vi "Weather Parse Test.vi"() -> ()   [LabVIEW 2020, in "CDM-Config.lvlib"] (continued)
    \"onset\": \"2025-12-03T00:00:00-08:00\",\n                \"expires\": \"2025-12-03T09:00:00-08:00\",\n                \"ends\": \"2025-12-03T09:00:00-08:00\",\n                \"status\": \"Actual\",\n                \"messageType\": \"Update\",\n                \"category\": \"Met\",\n                \"severity\": \"Minor\",\n                \"certainty\": \"Likely\",\n                \"urgency\": \"Expected\",\n                \"event\": \"Frost Advisory\",\n                \"sender\": \"w-nws.webmaster@noaa.gov\",\n                \"senderName\": \"NWS Eureka CA\",\n                \"headline\": \"Frost Advisory issued December 2 at 6:17PM PST until December 3 at 9:00AM PST by NWS Eureka CA\",\n                \"description\": \"* WHAT...Temperatures as low as 33 will result in frost formation.\\n\\n* WHERE...Humboldt Interior.\\n\\n* WHEN...From midnight tonight to 9 AM PST Wednesday.\\n\\n* IMPACTS...Frost could harm sensitive outdoor vegetation. Sensitive\\noutdoor plants may be killed if left uncovered.\\n\\n* ADDITIONAL DETAILS...Fog or low clouds may develop in some valleys\\nkeeping temperatures in the upper 30s.\",\n                \"instruction\": \"Take steps now to protect tender plants from the cold.\",\n                \"response\": \"Prepare\",\n                \"parameters\": {\n                    \"AWIPSidentifier\": [\n                        \"NPWEKA\"\n                    ],\n                    \"WMOidentifier\": [\n                        \"WWUS76 KEKA 030217\"\n                    ],\n                    \"NWSheadline\": [\n                        \"FROST ADVISORY REMAINS IN EFFECT FROM MIDNIGHT TONIGHT TO 9 AM PST WEDNESDAY\"\n                    ],\n                    \"BLOCKCHANNEL\": [\n                        \"EAS\",\n                        \"NWEM\",\n                        \"CMAS\"\n                    ],\n                    \"VTEC\": [\n                        \"/O.CON.KEKA.FR.Y.0037.251203T0800Z-251203T1700Z/\"\n                    ],\n                    \"eventEndingTime\": [\n                        \"2025-12-03T09:00:00-08:00\"\n                    ]\n                },\n                \"scope\": \"Public\",\n                \"code\": \"IPAWSv1.0\",\n                \"language\": \"en-US\",\n                \"web\": \"http://www.weather.gov\",\n                \"eventCode\": {\n                    \"SAME\": [\n                        \"NWS\"\n                    ],\n                    \"NationalWeatherService\": [\n                        \"FRY\"\n                    ]\n                }\n            }\n        },\n        {\n            \"id\": \"https://api.weather.gov/alerts/urn:oid:2.49.0.1.840.0.9a5af99817b4d9edcfcd61f0327d754f8de44e19.004.1\",\n            \"type\": \"Feature\",\n            \"geometry\": null,\n            \"properties\": {\n                \"@id\": \"https://api.weather.gov/alerts/urn:oid:2.49.0.1.840.0.9a5af99817b4d9edcfcd61f0327d754f8de44e19.004.1\",\n                \"@type\": \"wx:Alert\",\n                \"id\": \"urn:oid:2.49.0.1.840.0.9a5af99817b4d9edcfcd61f0327d754f8de44e19.004.1\",\n                \"areaDesc\": \"Southwestern Mendocino Interior; Southeastern Mendocino Interior\",\n                \"geocode\": {\n                    \"SAME\": [\n                        \"006045\"\n                    ],\n                    \"UGC\": [\n                        \"CAZ112\",\n                        \"CAZ113\"\n                    ]\n                },\n                \"affectedZones\": [\n                    \"https://api.weather.gov/zones/forecast/CAZ112\",\n                    \"https://api.weather.gov/zones/forecast/CAZ113\"\n                ],\n                \"references\": [\n                    {\n                        \"@id\": \"https://api.weather.gov/alerts/urn:oid:2.49.0.1.840.0.95406e8f32c287b077c961d659d14abba87dc6d0.003.1\",\n                        \"identifier\": \"urn:oid:2.49.0.1.840.0.95406e8f32c287b077c961d659d14abba87dc6d0.003.1\",\n                        \"sender\": \"w-nws.webmaster@noaa.gov\",\n                        \"sent\": \"2025-12-02T10:21:00-08:00\"\n                    },\n                    {\n                        \"@id\": \"https://api.weather.gov/alerts/urn:oid:2.49.0.1.840.0.572af28717b4d18ac951aaf092ab1eb478907437.004.1\",\n                        \"identifier\": \"urn:oid:2.49.0.1.840.0.572af28717b4d18ac951aaf092ab1eb478907437.004.1\",\n                        \"sender\": \"w-nws.webmaster@noaa.gov\",\n                        \"sent\": \"2025-12-02T10:26:00-08:00\"\n                    }\n                ],\n                \"sent\": \"2025-12-02T18:17:00-08:00\",\n                \"effective\": \"2025-12-02T18:17:00-08:00\",\n                \"onset\": \"2025-12-03T00:00:00-08:00\",\n                \"expires\": \"2025-12-03T09:00:00-08:00\",\n                \"ends\": \"2025-12-03T09:00:00-08:00\",\n                \"status\": \"Actual\",\n                \"messageType\": \"Update\",\n                \"category\": \"Met\",\n                \"severity\": \"Minor\",\n                \"certainty\": \"Likely\",\n                \"urgency\": \"Expected\",\n                \"event\": \"Frost Advisory\",\n                \"sender\": \"w-nws.webmaster@noaa.gov\",\n                \"senderName\": \"NWS Eureka CA\",\n                \"headline\": \"Frost Advisory issued December 2 at 6:17PM PST until December 3 at 9:00AM PST by NWS Eureka CA\",\n                \"description\": \"* WHAT...Temperatures as low as 34 will result in frost formation.\\n\\n* WHERE...Southern Mendocino Interior valleys.\\n\\n* WHEN...From midnight tonight to 9 AM PST Wednesday.\\n\\n* IMPACTS...Frost could harm sensitive outdoor vegetation. Sensitive\\noutdoor plants may be killed if left uncovered.\\n\\n* ADDITIONAL DETAILS...Fog or low clouds may develop in some valleys\\nkeeping temperatures in the upper 30s.\",\n                \"instruction\": \"Take steps now to protect tender plants from the cold.\",\n                \"response\": \"Prepare\",\n                \"parameters\": {\n                    \"AWIPSidentifier\": [\n                        \"NPWEKA\"\n                    ],\n                    \"WMOidentifier\": [\n                        \"WWUS76 KEKA 030217\"\n                    ],\n                    \"NWSheadline\": [\n                        \"FROST ADVISORY REMAINS IN EFFECT FROM MIDNIGHT TONIGHT TO 9 AM PST WEDNESDAY\"\n                    ],\n                    \"BLOCKCHANNEL\": [\n                        \"EAS\",\n                        \"NWEM\",\n                        \"CMAS\"\n                    ],\n                    \"VTEC\": [\n                        \"/O.CON.KEKA.FR.Y.0037.251203T0800Z-251203T1700Z/\"\n                    ],\n                    \"eventEndingTime\": [\n                        \"2025-12-03T09:00:00-08:00\"\n                    ]\n                },\n                \"scope\": \"Public\",\n                \"code\": \"IPAWSv1.0\",\n                \"language\": \"en-US\",\n                \"web\": \"http://www.weather.gov\",\n                \"eventCode\": {\n                    \"SAME\": [\n                        \"NWS\"\n                    ],\n                    \"NationalWeatherService\": [\n                        \"FRY\"\n                    ]\n                }\n            }\n        },\n        {\n            \"id\": \"https://api.weather.gov/alerts/urn:oid:2.49.0.1.840.0.9a5af99817b4d9edcfcd61f0327d754f8de44e19.001.1\",\n            \"type\": \"Feature\",\n            \"geometry\": null,\n            \"properties\": {\n                \"@id\": \"https://api.weather.gov/alerts/urn:oid:2.49.0.1.840.0.9a5af99817b4d9edcfcd61f0327d754f8de44e19.001.1\",\n                \"@type\": \"wx:Alert\",\n                \"id\": \"urn:oid:2.49.0.1.840.0.9a5af99817b4d9edcfcd61f0327d754f8de44e19.001.1\",\n                \"areaDesc\": \"Northern Humboldt Coast; Southwestern Humboldt\",\n                \"geocode\": {\n                    \"SAME\": [\n                        \"006023\"\n                    ],\n                    \"UGC\": [\n                        \"CAZ103\",\n                        \"CAZ104\"\n                    ]\n                },\n                \"affectedZones\": [\n                    \"https://api.weather.gov/zones/forecast/CAZ103\",\n                    \"https://api.weather.gov/zones/forecast/CAZ104\"\n                ],\n                \"references\": [\n                    {\n                        \"@id\": \"https://api.weather.gov/alerts/urn:oid:2.49.0.1.840.0.95406e8f32c287b077c961d659d14abba87dc6d0.001.1\",\n                        \"identifier\": \"urn:oid:2.49.0.1.840.0.95406e8f32c287b077c961d659d14abba87dc6d0.001.1\",\n                        \"sender\": \"w-nws.webmaster@noaa.gov\",\n                        \"sent\": \"2025-12-02T10:21:00-08:00\"\n                    },\n                    {\n                        \"@id\": \"https://api.weather.gov/alerts/urn:oid:2.49.0.1.840.0.572af28717b4d18ac951aaf092ab1eb478907437.002.1\",\n                        \"identifier\": \"urn:oid:2.49.0.1.840.0.572af28717b4d18ac951aaf092ab1eb478907437.002.1\",\n                        \"sender\": \"w-nws.webmaster@noaa.gov\",\n                        \"sent\": \"2025-12-02T10:26:00-08:00\"\n                    }\n                ],\n                \"sent\": \"2025-12-02T18:17:00-08:00\",\n                \"effective\": \"2025-12-02T18:17:00-08:00\",\n                \"onset\": \"2025-12-03T00:00:00-08:00\",\n                \"expires\": \"2025-12-03T09:00:00-08:00\",\n                \"ends\": \"2025-12-03T09:00:00-08:00\",\n                \"status\": \"Actual\",\n                \"messageType\": \"Update\",\n                \"category\": \"Met\",\n                \"severity\": \"Minor\",\n                \"certainty\": \"Likely\",\n                \"urgency\": \"Expected\",\n                \"event\": \"Frost Advisory\",\n                \"sender\": \"w-nws.webmaster@noaa.gov\",\n                \"senderName\": \"NWS Eureka CA\",\n                \"headline\": \"Frost Advisory issued December 2 at 6:17PM PST until December 3 at 9:00AM PST by NWS Eureka CA\",\n                \"description\": \"* WHAT...Temperatures as low as 34 will result in frost formation.\\n\\n* WHERE...Humboldt Coast.\\n\\n* WHEN...From midnight tonight to 9 AM PST Wednesday.\\n\\n* IMPACTS...Frost could harm sensitive outdoor vegetation. Sensitive\\noutdoor plants may be killed if left uncovered.\\n\\n* ADDITIONAL DETAILS...Coldest areas will be valleys that remain\\nclear and are away from the coast.\",\n                \"instruction\": \"Take steps now to protect tender plants from the cold.\",\n                \"response\": \"Prepare\",\n                \"parameters\": {\n                    \"AWIPSidentifier\": [\n                        \"NPWEKA\"\n                    ],\n                    \"WMOidentifier\": [\n                        \"WWUS76 KEKA 030217\"\n                    ],\n                    \"NWSheadline\": [\n                        \"FROST ADVISORY REMAINS IN EFFECT FROM MIDNIGHT TONIGHT TO 9 AM PST WEDNESDAY\"\n                    ],\n                    \"BLOCKCHANNEL\": [\n                        \"EAS\",\n                        \"NWEM\",\n                        \"CMAS\"\n                    ],\n                    \"VTEC\": [\n                        \"/O.CON.KEKA.FR.Y.0037.251203T0800Z-251203T1700Z/\"\n                    ],\n                    \"eventEndingTime\": [\n                        \"2025-12-03T09:00:00-08:00\"\n                    ]\n                },\n                \"scope\": \"Public\",\n                \"code\": \"IPAWSv1.0\",\n                \"language\": \"en-US\",\n                \"web\": \"http://www.weather.gov\",\n                \"eventCode\": {\n                    \"SAME\": [\n                        \"NWS\"\n                    ],\n                    \"NationalWeatherService\": [\n                        \"FRY\"\n                    ]\n                }\n            }\n        },\n        {\n            \"id\": \"https://api.weather.gov/alerts/urn:oid:2.49.0.1.840.0.9a5af99817b4d9edcfcd61f0327d754f8de44e19.003.1\",\n            \"type\": \"Feature\",\n            \"geometry\": null,\n            \"properties\": {\n                \"@id\": \"https://api.weather.gov/alerts/urn:oid:2.49.0.1.840.0.9a5af99817b4d9edcfcd61f0327d754f8de44e19.003.1\",\n                \"@type\": \"wx:Alert\",\n                \"id\": \"urn:oid:2.49.0.1.840.0.9a5af99817b4d9edcfcd61f0327d754f8de44e19.003.1\",\n                \"areaDesc\": \"Mendocino Coast\",\n                \"geocode\": {\n                    \"SAME\": [\n                        \"006045\"\n                    ],\n                    \"UGC\": [\n                        \"CAZ109\"\n                    ]\n                },\n                \"affectedZones\": [\n                    \"https://api.weather.gov/zones/forecast/CAZ109\"\n                ],\n                \"references\": [\n                    {\n                        \"@id\": \"https://api.weather.gov/alerts/urn:oid:2.49.0.1.840.0.95406e8f32c287b077c961d659d14abba87dc6d0.002.1\",\n                        \"identifier\": \"urn:oid:2.49.0.1.840.0.95406e8f32c287b077c961d659d14abba87dc6d0.002.1\",\n                        \"sender\": \"w-nws.webmaster@noaa.gov\",\n                        \"sent\": \"2025-12-02T10:21:00-08:00\"\n                    },\n                    {\n                        \"@id\": \"https://api.weather.gov/alerts/urn:oid:2.49.0.1.840.0.572af28717b4d18ac951aaf092ab1eb478907437.003.1\",\n                        \"identifier\": \"urn:oid:2.49.0.1.840.0.572af28717b4d18ac951aaf092ab1eb478907437.003.1\",\n                        \"sender\": \"w-nws.webmaster@noaa.gov\",\n                        \"sent\": \"2025-12-02T10:26:00-08:00\"\n                    }\n                ],\n                \"sent\": \"2025-12-02T18:17:00-08:00\",\n                \"effective\": \"2025-12-02T18:17:00-08:00\",\n                \"onset\": \"2025-12-03T00:00:00-08:00\",\n                \"expires\": \"2025-12-03T09:00:00-08:00\",\n                \"ends\": \"2025-12-03T09:00:00-08:00\",\n                \"status\": \"Actual\",\n                \"messageType\": \"Update\",\n                \"category\": \"Met\",\n                \"severity\": \"Minor\",\n                \"certainty\": \"Likely\",\n                \"urgency\": \"Expected\",\n                \"event\": \"Frost Advisory\",\n                \"sender\": \"w-nws.webmaster@noaa.gov\",\n                \"senderName\": \"NWS Eureka CA\",\n                \"headline\": \"Frost Advisory issued December 2 at 6:17PM PST until December 3 at 9:00AM PST by NWS Eureka CA\",\n                \"description\": \"* WHAT...Temperatures as low as 34 will result in frost formation.\\n\\n* WHERE...Mendocino Coast. The coldest areas will be just inland from\\nthe coast.\\n\\n* WHEN...From midnight tonight to 9 AM PST Wednesday.\\n\\n* IMPACTS...Frost could harm sensitive outdoor vegetation. Sensitive\\noutdoor plants may be killed if left uncovered.\",\n                \"instruction\": \"Take steps now to protect tender plants from the cold.\",\n                \"response\": \"Prepare\",\n                \"parameters\": {\n                    \"AWIPSidentifier\": [\n                        \"NPWEKA\"\n                    ],\n                    \"WMOidentifier\": [\n                        \"WWUS76 KEKA 030217\"\n                    ],\n                    \"NWSheadline\": [\n                        \"FROST ADVISORY REMAINS IN EFFECT FROM MIDNIGHT TONIGHT TO 9 AM PST WEDNESDAY\"\n                    ],\n                    \"BLOCKCHANNEL\": [\n                        \"EAS\",\n                        \"NWEM\",\n                        \"CMAS\"\n                    ],\n                    \"VTEC\": [\n                        \"/O.CON.KEKA.FR.Y.0037.251203T0800Z-251203T1700Z/\"\n                    ],\n                    \"eventEndingTime\": [\n                        \"2025-12-03T09:00:00-08:00\"\n                    ]\n                },\n                \"scope\": \"Public\",\n                \"code\": \"IPAWSv1.0\",\n                \"language\": \"en-US\",\n                \"web\": \"http://www.weather.gov\",\n                \"eventCode\": {\n                    \"SAME\": [\n                        \"NWS\"\n                    ],\n                    \"NationalWeatherService\": [\n                        \"FRY\"\n                    ]\n                }\n            }\n        },\n        {\n            \"id\": \"https://api.weather.gov/alerts/urn:oid:2.49.0.1.840.0.90d765b84bbb08e28d74a226f4e1f9e6e65de885.006.1\",\n            \"type\": \"Feature\",\n            \"geometry\": null,\n            \"properties\": {\n                \"@id\": \"https://api.weather.gov/alerts/urn:oid:2.49.0.1.840.0.90d765b84bbb08e28d74a226f4e1f9e6e65de885.006.1\",\n                \"@type\": \"wx:Alert\",\n                \"id\": \"urn:oid:2.49.0.1.840.0.90d765b84bbb08e28d74a226f4e1f9e6e65de885.006.1\",\n                \"areaDesc\": \"Cape Tolstoi to Cape Sarichef out to 15 NM\",\n                \"geocode\": {\n                    \"SAME\": [\n                        \"058754\"\n                    ],\n                    \"UGC\": [\n                        \"PKZ754\"\n                    ]\n                },\n                \"affectedZones\": [\n                    \"https://api.weather.gov/zones/forecast/PKZ754\"\n                ],\n                \"references\": [],\n                \"sent\": \"2025-12-02T16:08:00-09:00\",\n                \"effective\": \"2025-12-02T16:08:00-09:00\",\n                \"onset\": \"2025-12-03T05:00:00-09:00\",\n                \"expires\": \"2025-12-03T05:15:00-09:00\",\n                \"ends\": \"2025-12-04T05:00:00-09:00\",\n                \"status\": \"Actual\",\n                \"messageType\": \"Alert\",\n                \"category\": \"Met\",\n                \"severity\": \"Minor\",\n                \"certainty\": \"Likely\",\n                \"urgency\": \"Expected\",\n                \"event\": \"Small Craft Advisory\",\n                \"sender\": \"w-nws.webmaster@noaa.gov\",\n                \"senderName\": \"NWS Anchorage AK\",\n                \"headline\": \"Small Craft Advisory issued December 2 at 4:08PM AKST until December 4 at 5:00AM AKST by NWS Anchorage AK\",\n                \"description\": \"Coastal Waters Forecast for Southwest Alaska+Bristol Bay+The\\nAlaska Peninsula Waters and the Aleutian Islands up to 100 nm out.\\n\\nWind forecasts reflect the predominant speed and direction\\nexpected. Sea forecasts represent an average of the highest\\none-third of the combined wind wave and swell height.\\n\\n.TONIGHT...SE wind 30 kt. Seas 18 ft. Rain.\\n.WED...SE wind 25 kt. Seas 13 ft. Rain.\\n.WED NIGHT...SE wind 15 kt. Seas 11 ft. Rain.\\n.THU AND THU NIGHT...NE wind 15 kt. Seas 7 ft.\\n.FRI...N wind 25 kt. Seas 5 ft.\\n.SAT...NW wind 35 kt. Seas 6 ft.\\n.SUN...N wind 25 kt. Seas 5 ft.\",\n                \"instruction\": null,\n                \"response\": \"Avoid\",\n                \"parameters\": {\n                    \"AWIPSidentifier\": [\n                        \"CWFALU\"\n                    ],\n                    \"WMOidentifier\": [\n                        \"FZAK52 PAFC 030108\"\n                    ],\n                    \"NWSheadline\": [\n                        \"SMALL CRAFT ADVISORY THROUGH WEDNESDAY NIGHT\"\n                    ],\n                    \"BLOCKCHANNEL\": [\n                        \"EAS\",\n                        \"NWEM\",\n                        \"CMAS\"\n                    ],\n                    \"VTEC\": [\n                        \"/O.NEW.PAFC.SC.Y.9898.251203T1400Z-251204T1400Z/\"\n                    ],\n                    \"eventEndingTime\": [\n                        \"2025-12-04T05:00:00-09:00\"\n                    ]\n                },\n                \"scope\": \"Public\",\n                \"code\": \"IPAWSv1.0\",\n                \"language\": \"en-US\",\n                \"web\": \"http://www.weather.gov\",\n                \"eventCode\": {\n                    \"SAME\": [\n                        \"NWS\"\n                    ],\n                    \"NationalWeatherService\": [\n                        \"SCY\"\n                    ]\n                }\n            }\n        },\n        {\n            \"id\": \"https://api.weather.gov/alerts/urn:oid:2.49.0.1.840.0.90d765b84bbb08e28d74a226f4e1f9e6e65de885.003.1\",\n            \"type\": \"Feature\",\n            \"geometry\": null,\n            \"properties\": {\n                \"@id\": \"https://api.weather.gov/alerts/urn:oid:2.49.0.1.840.0.90d765b84bbb08e28d74a226f4e1f9e6e65de885.003.1\",\n                \"@type\": \"wx:Alert\",\n                \"id\": \"urn:oid:2.49.0.1.840.0.90d765b84bbb08e28d74a226f4e1f9e6e65de885.003.1\",\n                \"areaDesc\": \"Sitkinak to Castle Cape from 15 to 100 NM\",\n                \"geocode\": {\n                    \"SAME\": [\n                        \"058751\"\n                    ],\n                    \"UGC\": [\n                        \"PKZ751\"\n                    ]\n                },\n                \"affectedZones\": [\n                    \"https://api.weather.gov/zones/forecast/PKZ751\"\n                ],\n                \"references\": [],\n                \"sent\": \"2025-12-02T16:08:00-09:00\",\n                \"effective\": \"2025-12-02T16:08:00-09:00\",\n                \"onset\": \"2025-12-03T05:00:00-09:00\",\n                \"expires\": \"2025-12-03T05:15:00-09:00\",\n                \"ends\": \"2025-12-04T05:00:00-09:00\",\n                \"status\": \"Actual\",\n                \"messageType\": \"Alert\",\n                \"category\": \"Met\",\n                \"severity\": \"Minor\",\n                \"certainty\": \"Likely\",\n                \"urgency\": \"Expected\",\n                \"event\": \"Small Craft Advisory\",\n                \"sender\": \"w-nws.webmaster@noaa.gov\",\n                \"senderName\": \"NWS Anchorage AK\",\n                \"headline\": \"Small Craft Advisory issued December 2 at 4:08PM AKST until December 4 at 5:00AM AKST by NWS Anchorage AK\",\n                \"description\": \"Coastal Waters Forecast for Southwest Alaska+Bristol Bay+The\\nAlaska Peninsula Waters and the Aleutian Islands up to 100 nm out.\\n\\nWind forecasts reflect the predominant speed and direction\\nexpected. Sea forecasts represent an average of the highest\\none-third of the combined wind wave and swell height.\\n\\n.TONIGHT...SE wind 25 kt. Seas 17 ft.\\n.WED...S wind 20 kt. Seas 14 ft.\\n.WED NIGHT...S wind 20 kt. Seas 14 ft.\\n.THU...E wind 20 kt. Seas 12 ft.\\n.THU NIGHT...E wind 30 kt. Seas 10 ft.\\n.FRI THROUGH SAT...NW wind 35 kt. Seas 10 ft.\\n.SUN...N wind 25 kt. Seas 9 ft.\",\n                \"instruction\": null,\n                \"response\": \"Avoid\",\n                \"parameters\": {\n                    \"AWIPSidentifier\": [\n                        \"CWFALU\"\n                    ],\n                    \"WMOidentifier\": [\n                        \"FZAK52 PAFC 030108\"\n                    ],\n                    \"NWSheadline\": [\n                        \"SMALL CRAFT ADVISORY THROUGH WEDNESDAY NIGHT\"\n                    ],\n                    \"BLOCKCHANNEL\": [\n                        \"EAS\",\n                        \"NWEM\",\n                        \"CMAS\"\n                    ],\n                    \"VTEC\": [\n                        \"/O.NEW.PAFC.SC.Y.9895.251203T1400Z-251204T1400Z/\"\n                    ],\n                    \"eventEndingTime\": [\n                        \"2025-12-04T05:00:00-09:00\"\n                    ]\n                },\n                \"scope\": \"Public\",\n                \"code\": \"IPAWSv1.0\",\n                \"language\": \"en-US\",\n                \"web\": \"http://www.weather.gov\",\n                \"eventCode\": {\n                    \"SAME\": [\n                        \"NWS\"\n                    ],\n                    \"NationalWeatherService\": [\n                        \"SCY\"\n                    ]\n                }\n            }\n        },\n        {\n            \"id\": \"https://api.weather.gov/alerts/urn:oid:2.49.0.1.840.0.90d765b84bbb08e28d74a226f4e1f9e6e65de885.007.1\",\n            \"type\": \"Feature\",\n            \"geometry\": null,\n            \"properties\": {\n                \"@id\": \"https://api.weather.gov/alerts/urn:oid:2.49.0.1.840.0.90d765b84bbb08e28d74a226f4e1f9e6e65de885.007.1\",\n                \"@type\": \"wx:Alert\",\n                \"id\": \"urn:oid:2.49.0.1.840.0.90d765b84bbb08e28d74a226f4e1f9e6e65de885.007.1\",\n                \"areaDesc\": \"Cape Tolstoi to Cape Sarichef from 15 to 100 NM\",\n                \"geocode\": {\n                    \"SAME\": [\n                        \"058755\"\n                    ],\n                    \"UGC\": [\n                        \"PKZ755\"\n                    ]\n                },\n                \"affectedZones\": [\n                    \"https://api.weather.gov/zones/forecast/PKZ755\"\n                ],\n                \"references\": [],\n                \"sent\": \"2025-12-02T16:08:00-09:00\",\n                \"effective\": \"2025-12-02T16:08:00-09:00\",\n                \"onset\": \"2025-12-03T05:00:00-09:00\",\n                \"expires\": \"2025-12-03T05:15:00-09:00\",\n                \"ends\": \"2025-12-04T05:00:00-09:00\",\n                \"status\": \"Actual\",\n                \"messageType\": \"Alert\",\n                \"category\": \"Met\",\n                \"severity\": \"Minor\",\n                \"certainty\": \"Likely\",\n                \"urgency\": \"Expected\",\n                \"event\": \"Small Craft Advisory\",\n                \"sender\": \"w-nws.webmaster@noaa.gov\",\n                \"senderName\": \"NWS Anchorage AK\",\n                \"headline\": \"Small Craft Advisory issued December 2 at 4:08PM AKST until December 4 at 5:00AM AKST by NWS Anchorage AK\",\n                \"description\": \"Coastal Waters Forecast for Southwest Alaska+Bristol Bay+The\\nAlaska Peninsula Waters and the Aleutian Islands up to 100 nm out.\\n\\nWind forecasts reflect the predominant speed and direction\\nexpected. Sea forecasts represent an average of the highest\\none-third of the combined wind wave and swell height.\\n\\n.TONIGHT...SE wind 30 kt. Seas 21 ft. Rain.\\n.WED...SE wind 30 kt. Seas 18 ft. Rain.\\n.WED NIGHT...SE wind 25 kt. Seas 14 ft. Rain.\\n.THU...E wind 15 kt. Seas 11 ft.\\n.THU NIGHT...E wind 20 kt. Seas 7 ft.\\n.FRI...NW wind 20 kt. Seas 6 ft.\\n.SAT...NW wind 35 kt. Seas 13 ft.\\n.SUN...N wind 25 kt. Seas 10 ft.\",\n                \"instruction\": null,\n                \"response\": \"Avoid\",\n                \"parameters\": {\n                    \"AWIPSidentifier\": [\n                        \"CWFALU\"\n                    ],\n                    \"WMOidentifier\": [\n                        \"FZAK52 PAFC 030108\"\n                    ],\n                    \"NWSheadline\": [\n                        \"SMALL CRAFT ADVISORY THROUGH WEDNESDAY NIGHT\"\n                    ],\n                    \"BLOCKCHANNEL\": [\n                        \"EAS\",\n                        \"NWEM\",\n                        \"CMAS\"\n                    ],\n                    \"VTEC\": [\n                        \"/O.NEW.PAFC.SC.Y.9899.251203T1400Z-251204T1400Z/\"\n                    ],\n                    \"eventEndingTime\": [\n                        \"2025-12-04T05:00:00-09:00\"\n                    ]\n                },\n                \"scope\": \"Public\",\n                \"code\": \"IPAWSv1.0\",\n                \"language\": \"en-US\",\n                \"web\": \"http://www.weather.gov\",\n                \"eventCode\": {\n                    \"SAME\": [\n                        \"NWS\"\n                    ],\n                    \"NationalWeatherService\": [\n                        \"SCY\"\n                    ]\n                }\n            }\n        },\n        {\n            \"id\": \"https://api.weather.gov/alerts/urn:oid:2.49.0.1.840.0.90d765b84bbb08e28d74a226f4e1f9e6e65de885.016.1\",\n            \"type\": \"Feature\",\n            \"geometry\": null,\n            \"properties\": {\n                \"@id\": \"https://api.weather.gov/alerts/urn:oid:2.49.0.1.840.0.90d765b84bbb08e28d74a226f4e1f9e6e65de885.016.1\",\n                \"@type\": \"wx:Alert\",\n                \"id\": \"urn:oid:2.49.0.1.840.0.90d765b84bbb08e28d74a226f4e1f9e6e65de885.016.1\",\n                \"areaDesc\": \"Cape Sarichef to Nikoski Pacific Side from 15 to 85 NM\",\n                \"geocode\": {\n                    \"SAME\": [\n                        \"058774\"\n                    ],\n                    \"UGC\": [\n                        \"PKZ774\"\n                    ]\n                },\n                \"affectedZones\": [\n                    \"https://api.weather.gov/zones/forecast/PKZ774\"\n                ],\n                \"references\": [],\n                \"sent\": \"2025-12-02T16:08:00-09:00\",\n                \"effective\": \"2025-12-02T16:08:00-09:00\",\n                \"onset\": \"2025-12-03T05:00:00-09:00\",\n                \"expires\": \"2025-12-03T05:15:00-09:00\",\n                \"ends\": \"2025-12-04T05:00:00-09:00\",\n                \"status\": \"Actual\",\n                \"messageType\": \"Alert\",\n                \"category\": \"Met\",\n                \"severity\": \"Minor\",\n                \"certainty\": \"Likely\",\n                \"urgency\": \"Expected\",\n                \"event\": \"Small Craft Advisory\",\n                \"sender\": \"w-nws.webmaster@noaa.gov\",\n                \"senderName\": \"NWS Anchorage AK\",\n                \"headline\": \"Small Craft Advisory issued December 2 at 4:08PM AKST until December 4 at 5:00AM AKST by NWS Anchorage AK\",\n                \"description\": \"Coastal Waters Forecast for Southwest Alaska+Bristol Bay+The\\nAlaska Peninsula Waters and the Aleutian Islands up to 100 nm out.\\n\\nWind forecasts reflect the predominant speed and direction\\nexpected. Sea forecasts represent an average of the highest\\none-third of the combined wind wave and swell height.\\n\\n.TONIGHT...SE wind 30 kt. Seas 20 ft. Rain.\\n.WED...E wind 20 kt. Seas 18 ft. Rain.\\n.WED NIGHT...NE wind 20 kt. Seas 11 ft.\\n.THU...NE wind 20 kt. Seas 9 ft.\\n.THU NIGHT...E wind 15 kt. Seas 6 ft.\\n.FRI...SW wind 20 kt. Seas 5 ft.\\n.SAT THROUGH SUN...N wind 30 kt. Seas 11 ft.\",\n                \"instruction\": null,\n                \"response\": \"Avoid\",\n                \"parameters\": {\n                    \"AWIPSidentifier\": [\n                        \"CWFALU\"\n                    ],\n                    \"WMOidentifier\": [\n                        \"FZAK52 PAFC 030108\"\n                    ],\n                    \"NWSheadline\": [\n                        \"SMALL CRAFT ADVISORY THROUGH WEDNESDAY NIGHT\"\n                    ],\n                    \"BLOCKCHANNEL\": [\n                        \"EAS\",\n                        \"NWEM\",\n                        \"CMAS\"\n                    ],\n                    \"VTEC\": [\n                        \"/O.NEW.PAFC.SC.Y.9908.251203T1400Z-251204T1400Z/\"\n                    ],\n                    \"eventEndingTime\": [\n                        \"2025-12-04T05:00:00-09:00\"\n                    ]\n                },\n                \"scope\": \"Public\",\n                \"code\": \"IPAWSv1.0\",\n                \"language\": \"en-US\",\n                \"web\": \"http://www.weather.gov\",\n                \"eventCode\": {\n                    \"SAME\": [\n                        \"NWS\"\n                    ],\n                    \"NationalWeatherService\": [\n                        \"SCY\"\n                    ]\n                }\n            }\n        },\n        {\n            \"id\": \"https://api.weather.gov/alerts/urn:oid:2.49.0.1.840.0.90d765b84bbb08e28d74a226f4e1f9e6e65de885.025.1\",\n            \"type\": \"Feature\",\n            \"geometry\": null,\n            \"properties\": {\n                \"@id\": \"https://api.weather.gov/alerts/urn:oid:2.49.0.1.840.0.90d765b84bbb08e28d74a226f4e1f9e6e65de885.025.1\",\n                \"@type\": \"wx:Alert\",\n                \"id\": \"urn:oid:2.49.0.1.840.0.90d765b84bbb08e28d74a226f4e1f9e6e65de885.025.1\",\n                \"areaDesc\": \"Adak to Kiska Bering Side\",\n                \"geocode\": {\n                    \"SAME\": [\n                        \"058784\"\n                    ],\n                    \"UGC\": [\n                        \"PKZ784\"\n                    ]\n                },\n                \"affectedZones\": [\n                    \"https://api.weather.gov/zones/forecast/PKZ784\"\n                ],\n                \"references\": [],\n                \"sent\": \"2025-12-02T16:08:00-09:00\",\n                \"effective\": \"2025-12-02T16:08:00-09:00\",\n                \"onset\": \"2025-12-02T16:00:00-09:00\",\n                \"expires\": \"2025-12-03T05:15:00-09:00\",\n                \"ends\": \"2025-12-03T17:00:00-09:00\",\n                \"status\": \"Actual\",\n                \"messageType\": \"Alert\",\n                \"category\": \"Met\",\n                \"severity\": \"Moderate\",\n                \"certainty\": \"Likely\",\n                \"urgency\": \"Expected\",\n                \"event\": \"Gale Warning\",\n                \"sender\": \"w-nws.webmaster@noaa.gov\",\n                \"senderName\": \"NWS Anchorage AK\",\n                \"headline\": \"Gale Warning issued December 2 at 4:08PM AKST until December 3 at 5:00PM AKST by NWS Anchorage AK\",\n                \"description\": \"Coastal Waters Forecast for Southwest Alaska+Bristol Bay+The\\nAlaska Peninsula Waters and the Aleutian Islands up to 100 nm out.\\n\\nWind forecasts reflect the predominant speed and direction\\nexpected. Sea forecasts represent an average of the highest\\none-third of the combined wind wave and swell height.\\n\\n.TONIGHT...N wind 40 kt. Seas 28 ft.\\n.WED...N wind 40 kt. Seas 27 ft.\\n.WED NIGHT...NE wind 30 kt. Seas 20 ft.\\n.THU...E wind 30 kt. Seas 14 ft.\\n.THU NIGHT...SE wind 30 kt. Seas 10 ft.\\n.FRI...SW wind 20 kt. Seas 10 ft.\\n.SAT...NE wind 25 kt. Seas 10 ft.\\n.SUN...NE wind 30 kt. Seas 17 ft.\",\n                \"instruction\": null,\n                \"response\": \"Avoid\",\n                \"parameters\": {\n                    \"AWIPSidentifier\": [\n                        \"CWFALU\"\n                    ],\n                    \"WMOidentifier\": [\n                        \"FZAK52 PAFC 030108\"\n                    ],\n                    \"NWSheadline\": [\n                        \"GALE WARNING THROUGH WEDNESDAY\"\n                    ],\n                    \"BLOCKCHANNEL\": [\n                        \"EAS\",\n                        \"NWEM\",\n                        \"CMAS\"\n                    ],\n                    \"VTEC\": [\n                        \"/O.NEW.PAFC.GL.W.9917.251203T0100Z-251204T0200Z/\"\n                    ],\n                    \"eventEndingTime\": [\n                        \"2025-12-03T17:00:00-09:00\"\n                    ]\n                },\n                \"scope\": \"Public\",\n                \"code\": \"IPAWSv1.0\",\n                \"language\": \"en-US\",\n                \"web\": \"http://www.weather.gov\",\n                \"eventCode\": {\n                    \"SAME\": [\n                        \"NWS\"\n                    ],\n                    \"NationalWeatherService\": [\n                        \"GLW\"\n                    ]\n                }\n            }\n        },\n        {\n            \"id\": \"https://api.weather.gov/alerts/urn:oid:2.49.0.1.840.0.90d765b84bbb08e28d74a226f4e1f9e6e65de885.002.1\",\n            \"type\": \"Feature\",\n            \"geometry\": null,\n            \"properties\": {\n                \"@id\": \"https://api.weather.gov/alerts/urn:oid:2.49.0.1.840.0.90d765b84bbb08e28d74a226f4e1f9e6e65de885.002.1\",\n                \"@type\": \"wx:Alert\",\n                \"id\": \"urn:oid:2.49.0.1.840.0.90d765b84bbb08e28d74a226f4e1f9e6e65de885.002.1\",\n                \"areaDesc\": \"Sitkinak to Castle Cape out to 15 NM\",\n                \"geocode\": {\n                    \"SAME\": [\n                        \"058750\"\n                    ],\n                    \"UGC\": [\n                        \"PKZ750\"\n                    ]\n                },\n                \"affectedZones\": [\n                    \"https://api.weather.gov/zones/forecast/PKZ750\"\n                ],\n                \"references\": [],\n                \"sent\": \"2025-12-02T16:08:00-09:00\",\n                \"effective\": \"2025-12-02T16:08:00-09:00\",\n                \"onset\": \"2025-12-03T05:00:00-09:00\",\n                \"expires\": \"2025-12-03T05:15:00-09:00\",\n                \"ends\": \"2025-12-04T05:00:00-09:00\",\n                \"status\": \"Actual\",\n                \"messageType\": \"Alert\",\n                \"category\": \"Met\",\n                \"severity\": \"Minor\",\n                \"certainty\": \"Likely\",\n                \"urgency\": \"Expected\",\n                \"event\": \"Small Craft Advisory\",\n                \"sender\": \"w-nws.webmaster@noaa.gov\",\n                \"senderName\": \"NWS Anchorage AK\",\n                \"headline\": \"Small Craft Advisory issued December 2 at 4:08PM AKST until December 4 at 5:00AM AKST by NWS Anchorage AK\",\n                \"description\": \"Coastal Waters Forecast for Southwest Alaska+Bristol Bay+The\\nAlaska Peninsula Waters and the Aleutian Islands up to 100 nm out.\\n\\nWind forecasts reflect the predominant speed and direction\\nexpected. Sea forecasts represent an average of the highest\\none-third of the combined wind wave and swell height.\\n\\n.TONIGHT...SE wind 25 kt. Seas 13 ft. Rain.\\n.WED...SE wind 20 kt. Seas 10 ft. Rain.\\n.WED NIGHT...SE wind 20 kt. Seas 10 ft. Rain.\\n.THU...E wind 20 kt. Seas 9 ft.\\n.THU NIGHT...NE wind 25 kt. Seas 7 ft.\\n.FRI THROUGH SAT...NW wind 35 kt. Seas 7 ft.\\n.SUN...NW wind 25 kt. Seas 5 ft.\",\n                \"instruction\": null,\n                \"response\": \"Avoid\",\n                \"parameters\": {\n                    \"AWIPSidentifier\": [\n                        \"CWFALU\"\n                    ],\n                    \"WMOidentifier\": [\n                        \"FZAK52 PAFC 030108\"\n                    ],\n                    \"NWSheadline\": [\n                        \"SMALL CRAFT ADVISORY THROUGH WEDNESDAY NIGHT\"\n                    ],\n                    \"BLOCKCHANNEL\": [\n                        \"EAS\",\n                        \"NWEM\",\n                        \"CMAS\"\n                    ],\n                    \"VTEC\": [\n                        \"/O.NEW.PAFC.SC.Y.9894.251203T1400Z-251204T1400Z/\"\n                    ],\n                    \"eventEndingTime\": [\n                        \"2025-12-04T05:00:00-09:00\"\n                    ]\n                },\n                \"scope\": \"Public\",\n                \"code\": \"IPAWSv1.0\",\n                \"language\": \"en-US\",\n                \"web\": \"http://www.weather.gov\",\n                \"eventCode\": {\n                    \"SAME\": [\n                        \"NWS\"\n                    ],\n                    \"NationalWeatherService\": [\n                        \"SCY\"\n                    ]\n                }\n            }\n        },\n        {\n            \"id\": \"https://api.weather.gov/alerts/urn:oid:2.49.0.1.840.0.90d765b84bbb08e28d74a226f4e1f9e6e65de885.030.1\",\n            \"type\": \"Feature\",\n            \"geometry\": null,\n            \"properties\": {\n                \"@id\": \"https://api.weather.gov/alerts/urn:oid:2.49.0.1.840.0.90d765b84bbb08e28d74a226f4e1f9e6e65de885.030.1\",\n                \"@type\": \"wx:Alert\",\n                \"id\": \"urn:oid:2.49.0.1.840.0.90d765b84bbb08e28d74a226f4e1f9e6e65de885.030.1\",\n                \"areaDesc\": \"Bristol Bay greater than 15 NM\",\n                \"geocode\": {\n                    \"SAME\": [\n                        \"058760\"\n                    ],\n                    \"UGC\": [\n                        \"PKZ760\"\n                    ]\n                },\n                \"affectedZones\": [\n                    \"https://api.weather.gov/zones/forecast/PKZ760\"\n                ],\n                \"references\": [],\n                \"sent\": \"2025-12-02T16:08:00-09:00\",\n                \"effective\": \"2025-12-02T16:08:00-09:00\",\n                \"onset\": \"2025-12-03T05:00:00-09:00\",\n                \"expires\": \"2025-12-03T05:15:00-09:00\",\n                \"ends\": \"2025-12-04T05:00:00-09:00\",\n                \"status\": \"Actual\",\n                \"messageType\": \"Alert\",\n                \"category\": \"Met\",\n                \"severity\": \"Minor\",\n                \"certainty\": \"Likely\",\n                \"urgency\": \"Expected\",\n                \"event\": \"Small Craft Advisory\",\n                \"sender\": \"w-nws.webmaster@noaa.gov\",\n                \"senderName\": \"NWS Anchorage AK\",\n                \"headline\": \"Small Craft Advisory issued December 2 at 4:08PM AKST until December 4 at 5:00AM AKST by NWS Anchorage AK\",\n                \"description\": \"Coastal Waters Forecast for Southwest Alaska+Bristol Bay+The\\nAlaska Peninsula Waters and the Aleutian Islands up to 100 nm out.\\n\\nWind forecasts reflect the predominant speed and direction\\nexpected. Sea forecasts represent an average of the highest\\none-third of the combined wind wave and swell height.\\n\\n.TONIGHT...SE wind 25 kt. Seas 6 ft.\\n.WED...E wind 25 kt. Seas 6 ft.\\n.WED NIGHT...E wind 25 kt. Seas 5 ft. Rain.\\n.THU AND THU NIGHT...NE wind 25 kt. Seas 6 ft.\\n.FRI THROUGH SUN...NE wind 30 kt. Seas 8 ft.\",\n                \"instruction\": null,\n                \"response\": \"Avoid\",\n                \"parameters\": {\n                    \"AWIPSidentifier\": [\n                        \"CWFALU\"\n                    ],\n                    \"WMOidentifier\": [\n                        \"FZAK52 PAFC 030108\"\n                    ],\n                    \"NWSheadline\": [\n                        \"SMALL CRAFT ADVISORY THROUGH WEDNESDAY NIGHT\"\n                    ],\n                    \"BLOCKCHANNEL\": [\n                        \"EAS\",\n                        \"NWEM\",\n                        \"CMAS\"\n                    ],\n                    \"VTEC\": [\n                        \"/O.NEW.PAFC.SC.Y.9922.251203T1400Z-251204T1400Z/\"\n                    ],\n                    \"eventEndingTime\": [\n                        \"2025-12-04T05:00:00-09:00\"\n                    ]\n                },\n                \"scope\": \"Public\",\n                \"code\": \"IPAWSv1.0\",\n                \"language\": \"en-US\",\n                \"web\": \"http://www.weather.gov\",\n                \"eventCode\": {\n                    \"SAME\": [\n                        \"NWS\"\n                    ],\n                    \"NationalWeatherService\": [\n                        \"SCY\"\n                    ]\n                }\n            }\n        },\n        {\n            \"id\": \"https://api.weather.gov/alerts/urn:oid:2.49.0.1.840.0.90d765b84bbb08e28d74a226f4e1f9e6e65de885.027.1\",\n            \"type\": \"Feature\",\n            \"geometry\": null,\n            \"properties\": {\n                \"@id\": \"https://api.weather.gov/alerts/urn:oid:2.49.0.1.840.0.90d765b84bbb08e28d74a226f4e1f9e6e65de885.027.1\",\n                \"@type\": \"wx:Alert\",\n                \"id\": \"urn:oid:2.49.0.1.840.0.90d765b84bbb08e28d74a226f4e1f9e6e65de885.027.1\",\n                \"areaDesc\": \"Kiska to Attu Bering Side\",\n                \"geocode\": {\n                    \"SAME\": [\n                        \"058786\"\n                    ],\n                    \"UGC\": [\n                        \"PKZ786\"\n                    ]\n                },\n                \"affectedZones\": [\n                    \"https://api.weather.gov/zones/forecast/PKZ786\"\n                ],\n                \"references\": [],\n                \"sent\": \"2025-12-02T16:08:00-09:00\",\n                \"effective\": \"2025-12-02T16:08:00-09:00\",\n                \"onset\": \"2025-12-03T17:00:00-09:00\",\n                \"expires\": \"2025-12-03T05:15:00-09:00\",\n                \"ends\": \"2025-12-04T05:00:00-09:00\",\n                \"status\": \"Actual\",\n                \"messageType\": \"Alert\",\n                \"category\": \"Met\",\n                \"severity\": \"Moderate\",\n                \"certainty\": \"Likely\",\n                \"urgency\": \"Expected\",\n                \"event\": \"Gale Warning\",\n                \"sender\": \"w-nws.webmaster@noaa.gov\",\n                \"senderName\": \"NWS Anchorage AK\",\n                \"headline\": \"Gale Warning issued December 2 at 4:08PM AKST until December 4 at 5:00AM AKST by NWS Anchorage AK\",\n                \"description\": \"Coastal Waters Forecast for Southwest Alaska+Bristol Bay+The\\nAlaska Peninsula Waters and the Aleutian Islands up to 100 nm out.\\n\\nWind forecasts reflect the predominant speed and direction\\nexpected. Sea forecasts represent an average of the highest\\none-third of the combined wind wave and swell height.\\n\\n.TONIGHT...N wind 30 kt. Seas 22 ft.\\n.WED...NE wind 25 kt. Seas 20 ft.\\n.WED NIGHT...E wind 30 kt becoming SE 40 kt after midnight. Seas\\n16 ft.\\n.THU...SE wind 45 kt. Seas 19 ft.\\n.THU NIGHT...SE wind 40 kt. Seas 20 ft.\\n.FRI...NW wind 30 kt. Seas 15 ft.\\n.SAT THROUGH SUN...NE wind 25 kt. Seas 12 ft.\",\n                \"instruction\": null,\n                \"response\": \"Avoid\",\n                \"parameters\": {\n                    \"AWIPSidentifier\": [\n                        \"CWFALU\"\n                    ],\n                    \"WMOidentifier\": [\n                        \"FZAK52 PAFC 030108\"\n                    ],\n                    \"NWSheadline\": [\n                        \"GALE WARNING WEDNESDAY NIGHT\"\n                    ],\n                    \"BLOCKCHANNEL\": [\n                        \"EAS\",\n                        \"NWEM\",\n                        \"CMAS\"\n                    ],\n                    \"VTEC\": [\n                        \"/O.NEW.PAFC.GL.W.9919.251204T0200Z-251204T1400Z/\"\n                    ],\n                    \"eventEndingTime\": [\n                        \"2025-12-04T05:00:00-09:00\"\n                    ]\n                },\n                \"scope\": \"Public\",\n                \"code\": \"IPAWSv1.0\",\n                \"language\": \"en-US\",\n                \"web\": \"http://www.weather.gov\",\n                \"eventCode\": {\n                    \"SAME\": [\n                        \"NWS\"\n                    ],\n                    \"NationalWeatherService\": [\n                        \"GLW\"\n                    ]\n                }\n            }\n        },\n        {\n            \"id\": \"https://api.weather.gov/alerts/urn:oid:2.49.0.1.840.0.90d765b84bbb08e28d74a226f4e1f9e6e65de885.028.1\",\n            \"type\": \"Feature\",\n            \"geometry\": null,\n            \"properties\": {\n                \"@id\": \"https://api.weather.gov/alerts/urn:oid:2.49.0.1.840.0.90d765b84bbb08e28d74a226f4e1f9e6e65de885.028.1\",\n                \"@type\": \"wx:Alert\",\n                \"id\": \"urn:oid:2.49.0.1.840.0.90d765b84bbb08e28d74a226f4e1f9e6e65de885.028.1\",\n                \"areaDesc\": \"Kiska to Attu Pacific Side\",\n                \"geocode\": {\n                    \"SAME\": [\n                        \"058787\"\n                    ],\n                    \"UGC\": [\n                        \"PKZ787\"\n                    ]\n                },\n                \"affectedZones\": [\n                    \"https://api.weather.gov/zones/forecast/PKZ787\"\n                ],\n                \"references\": [],\n                \"sent\": \"2025-12-02T16:08:00-09:00\",\n                \"effective\": \"2025-12-02T16:08:00-09:00\",\n                \"onset\": \"2025-12-03T17:00:00-09:00\",\n                \"expires\": \"2025-12-03T05:15:00-09:00\",\n                \"ends\": \"2025-12-04T05:00:00-09:00\",\n                \"status\": \"Actual\",\n                \"messageType\": \"Alert\",\n                \"category\": \"Met\",\n                \"severity\": \"Moderate\",\n                \"certainty\": \"Likely\",\n                \"urgency\": \"Expected\",\n                \"event\": \"Gale Warning\",\n                \"sender\": \"w-nws.webmaster@noaa.gov\",\n                \"senderName\": \"NWS Anchorage AK\",\n                \"headline\": \"Gale Warning issued December 2 at 4:08PM AKST until December 4 at 5:00AM AKST by NWS Anchorage AK\",\n                \"description\": \"Coastal Waters Forecast for Southwest Alaska+Bristol Bay+The\\nAlaska Peninsula Waters and the Aleutian Islands up to 100 nm out.\\n\\nWind forecasts reflect the predominant speed and direction\\nexpected. Sea forecasts represent an average of the highest\\none-third of the combined wind wave and swell height.\\n\\n.TONIGHT...N wind 30 kt. Seas 19 ft.\\n.WED...NE wind 25 kt. Seas 17 ft.\\n.WED NIGHT...E wind 30 kt becoming SE 45 kt after midnight. Seas\\n14 ft.\\n.THU...SE wind 50 kt. Seas 22 ft.\\n.THU NIGHT...SW wind 40 kt. Seas 22 ft.\\n.FRI...W wind 30 kt. Seas 17 ft.\\n.SAT THROUGH SUN...NE wind 25 kt. Seas 12 ft.\",\n                \"instruction\": null,\n                \"response\": \"Avoid\",\n                \"parameters\": {\n                    \"AWIPSidentifier\": [\n                        \"CWFALU\"\n                    ],\n                    \"WMOidentifier\": [\n                        \"FZAK52 PAFC 030108\"\n                    ],\n                    \"NWSheadline\": [\n                        \"GALE WARNING WEDNESDAY NIGHT\"\n                    ],\n                    \"BLOCKCHANNEL\": [\n                        \"EAS\",\n                        \"NWEM\",\n                        \"CMAS\"\n                    ],\n                    \"VTEC\": [\n                        \"/O.NEW.PAFC.GL.W.9920.251204T0200Z-251204T1400Z/\"\n                    ],\n                    \"eventEndingTime\": [\n                        \"2025-12-04T05:00:00-09:00\"\n                    ]\n                },\n                \"scope\": \"Public\",\n                \"code\": \"IPAWSv1.0\",\n                \"language\": \"en-US\",\n                \"web\": \"http://www.weather.gov\",\n                \"eventCode\": {\n                    \"SAME\": [\n                        \"NWS\"\n                    ],\n                    \"NationalWeatherService\": [\n                        \"GLW\"\n                    ]\n                }\n            }\n        },\n        {\n            \"id\": \"https://api.weather.gov/alerts/urn:oid:2.49.0.1.840.0.90d765b84bbb08e28d74a226f4e1f9e6e65de885.024.1\",\n            \"type\": \"Feature\",\n            \"geometry\": null,\n            \"properties\": {\n                \"@id\": \"https://api.weather.gov/alerts/urn:oid:2.49.0.1.840.0.90d765b84bbb08e28d74a226f4e1f9e6e65de885.024.1\",\n                \"@type\": \"wx:Alert\",\n                \"id\": \"urn:oid:2.49.0.1.840.0.90d765b84bbb08e28d74a226f4e1f9e6e65de885.024.1\",\n                \"areaDesc\": \"Seguam to Adak Pacific Side from 15 to 75 NM\",\n                \"geocode\": {\n                    \"SAME\": [\n                        \"058783\"\n                    ],\n                    \"UGC\": [\n                        \"PKZ783\"\n                    ]\n                },\n                \"affectedZones\": [\n                    \"https://api.weather.gov/zones/forecast/PKZ783\"\n                ],\n                \"references\": [],\n                \"sent\": \"2025-12-02T16:08:00-09:00\",\n                \"effective\": \"2025-12-02T16:08:00-09:00\",\n                \"onset\": \"2025-12-03T05:00:00-09:00\",\n                \"expires\": \"2025-12-03T05:15:00-09:00\",\n                \"ends\": \"2025-12-04T05:00:00-09:00\",\n                \"status\": \"Actual\",\n                \"messageType\": \"Alert\",\n                \"category\": \"Met\",\n                \"severity\": \"Moderate\",\n                \"certainty\": \"Likely\",\n                \"urgency\": \"Expected\",\n                \"event\": \"Gale Warning\",\n                \"sender\": \"w-nws.webmaster@noaa.gov\",\n                \"senderName\": \"NWS Anchorage AK\",\n                \"headline\": \"Gale Warning issued December 2 at 4:08PM AKST until December 4 at 5:00AM AKST by NWS Anchorage AK\",\n                \"description\": \"Coastal Waters Forecast for Southwest Alaska+Bristol Bay+The\\nAlaska Peninsula Waters and the Aleutian Islands up to 100 nm out.\\n\\nWind forecasts reflect the predominant speed and direction\\nexpected. Sea forecasts represent an average of the highest\\none-third of the combined wind wave and swell height.\\n\\n.TONIGHT...N wind 45 kt. Seas 20 ft.\\n.WED...N wind 35 kt. Seas 16 ft.\\n.WED NIGHT...N wind 35 kt. Seas 14 ft.\\n.THU...N wind 30 kt. Seas 11 ft.\\n.THU NIGHT...NE wind 15 kt. Seas 7 ft.\\n.FRI...NE wind 20 kt. Seas 11 ft.\\n.SAT...N wind 25 kt. Seas 11 ft.\\n.SUN...N wind 35 kt. Seas 16 ft.\",\n                \"instruction\": null,\n                \"response\": \"Avoid\",\n                \"parameters\": {\n                    \"AWIPSidentifier\": [\n                        \"CWFALU\"\n                    ],\n                    \"WMOidentifier\": [\n                        \"FZAK52 PAFC 030108\"\n                    ],\n                    \"NWSheadline\": [\n                        \"GALE WARNING THROUGH WEDNESDAY NIGHT\"\n                    ],\n                    \"BLOCKCHANNEL\": [\n                        \"EAS\",\n                        \"NWEM\",\n                        \"CMAS\"\n                    ],\n                    \"VTEC\": [\n                        \"/O.NEW.PAFC.GL.W.9916.251203T1400Z-251204T1400Z/\"\n                    ],\n                    \"eventEndingTime\": [\n                        \"2025-12-04T05:00:00-09:00\"\n                    ]\n                },\n                \"scope\": \"Public\",\n                \"code\": \"IPAWSv1.0\",\n                \"language\": \"en-US\",\n                \"web\": \"http://www.weather.gov\",\n                \"eventCode\": {\n                    \"SAME\": [\n                        \"NWS\"\n                    ],\n                    \"NationalWeatherService\": [\n                        \"GLW\"\n                    ]\n                }\n            }\n        },\n        {\n            \"id\": \"https://api.weather.gov/alerts/urn:oid:2.49.0.1.840.0.90d765b84bbb08e28d74a226f4e1f9e6e65de885.033.1\",\n            \"type\": \"Feature\",\n            \"geometry\": null,\n            \"properties\": {\n                \"@id\": \"https://api.weather.gov/alerts/urn:oid:2.49.0.1.840.0.90d765b84bbb08e28d74a226f4e1f9e6e65de885.033.1\",\n                \"@type\": \"wx:Alert\",\n                \"id\": \"urn:oid:2.49.0.1.840.0.90d765b84bbb08e28d74a226f4e1f9e6e65de885.033.1\",\n                \"areaDesc\": \"Kuskokwim Delta and Etolin Strait out to 15 NM\",\n                \"geocode\": {\n                    \"SAME\": [\n                        \"058763\"\n                    ],\n                    \"UGC\": [\n                        \"PKZ763\"\n                    ]\n                },\n                \"affectedZones\": [\n                    \"https://api.weather.gov/zones/forecast/PKZ763\"\n                ],\n                \"references\": [],\n                \"sent\": \"2025-12-02T16:08:00-09:00\",\n                \"effective\": \"2025-12-02T16:08:00-09:00\",\n                \"onset\": \"2025-12-03T05:00:00-09:00\",\n                \"expires\": \"2025-12-03T05:15:00-09:00\",\n                \"ends\": \"2025-12-04T05:00:00-09:00\",\n                \"status\": \"Actual\",\n                \"messageType\": \"Alert\",\n                \"category\": \"Met\",\n                \"severity\": \"Minor\",\n                \"certainty\": \"Likely\",\n                \"urgency\": \"Expected\",\n                \"event\": \"Small Craft Advisory\",\n                \"sender\": \"w-nws.webmaster@noaa.gov\",\n                \"senderName\": \"NWS Anchorage AK\",\n                \"headline\": \"Small Craft Advisory issued December 2 at 4:08PM AKST until December 4 at 5:00AM AKST by NWS Anchorage AK\",\n                \"description\": \"Coastal Waters Forecast for Southwest Alaska+Bristol Bay+The\\nAlaska Peninsula Waters and the Aleutian Islands up to 100 nm out.\\n\\nWind forecasts reflect the predominant speed and direction\\nexpected. Sea forecasts represent an average of the highest\\none-third of the combined wind wave and swell height.\\n\\n.TONIGHT...NE wind 30 kt. Seas in ice free waters 4 ft. Freezing\\nspray.\\n.WED...NE wind 25 kt. Seas in ice free waters 4 ft. Freezing spray.\\n.WED NIGHT...N wind 30 kt. Seas in ice free waters 4 ft. Freezing\\nspray.\\n.THU AND THU NIGHT...NE wind 25 kt. Seas in ice free waters 3 ft.\\n.FRI...N wind 35 kt. Seas in ice free waters 4 ft.\\n.SAT...N wind 45 kt. Seas in ice free waters 7 ft.\\n.SUN...N wind 40 kt. Seas in ice free waters 6 ft.\",\n                \"instruction\": null,\n                \"response\": \"Avoid\",\n                \"parameters\": {\n                    \"AWIPSidentifier\": [\n                        \"CWFALU\"\n                    ],\n                    \"WMOidentifier\": [\n                        \"FZAK52 PAFC 030108\"\n                    ],\n                    \"NWSheadline\": [\n                        \"SMALL CRAFT ADVISORY THROUGH WEDNESDAY NIGHT\"\n                    ],\n                    \"BLOCKCHANNEL\": [\n                        \"EAS\",\n                        \"NWEM\",\n                        \"CMAS\"\n                    ],\n                    \"VTEC\": [\n                        \"/O.NEW.PAFC.SC.Y.9925.251203T1400Z-251204T1400Z/\"\n                    ],\n                    \"eventEndingTime\": [\n                        \"2025-12-04T05:00:00-09:00\"\n                    ]\n                },\n                \"scope\": \"Public\",\n                \"code\": \"IPAWSv1.0\",\n                \"language\": \"en-US\",\n                \"web\": \"http://www.weather.gov\",\n                \"eventCode\": {\n                    \"SAME\": [\n                        \"NWS\"\n                    ],\n                    \"NationalWeatherService\": [\n                        \"SCY\"\n                    ]\n                }\n            }\n        },\n        {\n            \"id\": \"https://api.weather.gov/alerts/urn:oid:2.49.0.1.840.0.90d765b84bbb08e28d74a226f4e1f9e6e65de885.015.1\",\n            \"type\": \"Feature\",\n            \"geometry\": null,\n            \"properties\": {\n                \"@id\": \"https://api.weather.gov/alerts/urn:oid:2.49.0.1.840.0.90d765b84bbb08e28d74a226f4e1f9e6e65de885.015.1\",\n                \"@type\": \"wx:Alert\",\n                \"id\": \"urn:oid:2.49.0.1.840.0.90d765b84bbb08e28d74a226f4e1f9e6e65de885.015.1\",\n                \"areaDesc\": \"Cape Sarichef to Nikoski Pacific Side out to 15 NM\",\n                \"geocode\": {\n                    \"SAME\": [\n                        \"058773\"\n                    ]
